vi "GPIB Send Receive_VISA.vi"(1 "RDY max wait, ms":u32=500, 4 "RDY when up":bool=TRUE, 5 "Data ready bit (-1 - ignore)":i32=-1, 6 "Read terminator":i16, 7 "Delay, ms":u32, 8 "error in (no error)":errorcluster, 9 "Receive count":i32=256, 10 "data string in":string, 11 "VISA resource name":refnum<visa-resource-name>) -> (0 "error out":errorcluster, 2 "data string out":string, 3 "VISA resource name out":refnum<visa-resource-name>)   [LabVIEW 2015]
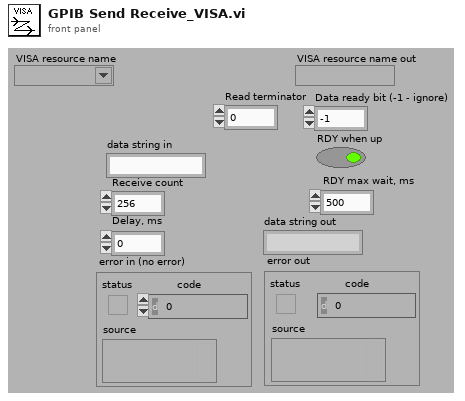
[diagram p1: front panel]
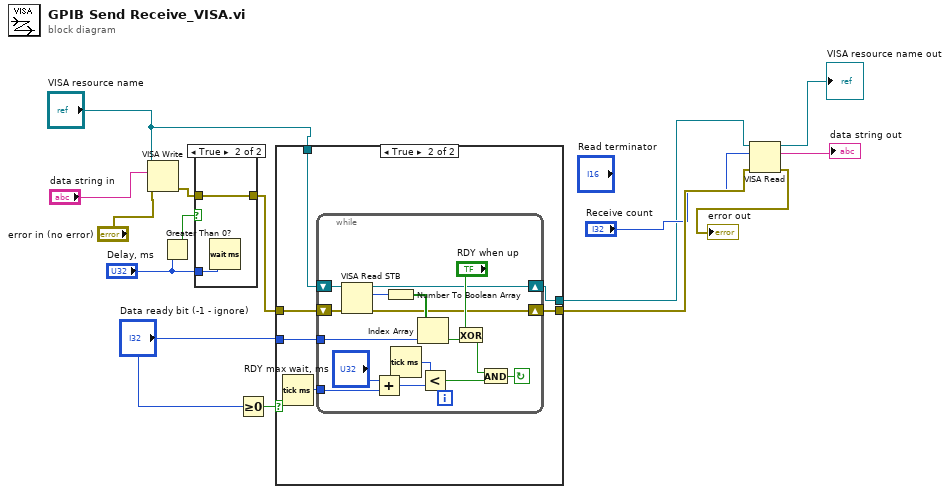
[diagram p0: block diagram]
diagram:
  n1 = VISA Write(VISA resource name="VISA resource name", write buffer="data string in", error in (no error)="error in (no error)") -> (error out=w10:errorcluster)  [unwired: 2 out]
  n2 = Greater Than 0?(x="Delay, ms") -> (x > 0?=w15:bool)
  n3 = case shown="True" w15 {
    tunnel: w10 -> [w16 w17]
    tunnel: [w16 w17] -> w12
    tunnel: "Delay, ms" -> [_ w18]
    frame False {
    }
    frame True {
      n4 = Wait (ms)(milliseconds to wait=w18) -> ()  [unwired: 1 out]
    }
  }
  n5 = Greater Or Equal To 0?(x="Data ready bit (-1 - ignore)") -> (x >= 0?=w13:bool)
  n6 = case shown="True" w13 {
    tunnel: "VISA resource name" -> [w19 w25]
    tunnel: w12 -> [w20 w24]
    tunnel: "Data ready bit (-1 - ignore)" -> [_ w23]
    tunnel: [w20 w22] -> w7
    tunnel: [w19 w21] -> w1
    frame False {
    }
    frame True {
      n7 = Tick Count (ms)() -> (millisecond timer value=w26:u32)
      n8 = while {
        shift-right: [w28] -> w22
        shift-left: w24 -> [w29]
        tunnel: w26 -> [w39]
        tunnel: w23 -> [w35]
        shift-right: [w27] -> w21
        shift-left: w25 -> [w31]
        stop <- w42 continue-if-true
        n9 = VISA Read STB(8:w29, 11:w31) -> (0:w28:errorcluster, 2:w30:u16, 3:w27:refnum<visa-resource-name>)
        n10 = Add(x="RDY max wait, ms", y=w39) -> (x+y=w40:u32)
        n11 = Number To Boolean Array(number=w30) -> (Boolean array=w37:bool[])
        n12 = Tick Count (ms)() -> (millisecond timer value=w38:u32)
        n13 = Index Array(array=w37, index=w35) -> (element=w34:bool)
        n14 = Less?(x=w38, y=w40) -> (x < y?=w41:bool)
        n15 = Exclusive Or(1:w34, 2:"RDY when up") -> (0:w33:bool)
        n16 = And(x=w33, y=w41) -> (x .and. y?=w42:bool)
      }
    }
  }
  n17 = VISA Read(VISA resource name=w1, byte count="Receive count", error in (no error)=w7) -> (VISA resource name out=→"VISA resource name out":refnum<visa-resource-name>, read buffer=→"data string out":string, error out=→"error out":errorcluster)  [unwired: 1 out]
